vi "save_file.vi"(4 "offset":dbl, 5 "write OME header? (T)":bool=TRUE, 6 "multiplication factor":dbl=1.0, 7 "path":path, 8 "error in (no error)":errorcluster, 10 "ImageCollection in":refnum<class "ImageCollection.lvclass">, 11 "DataCollectionDL090215 in":refnum<class "DataCollectionMG091001IntrinsicImaging.lvclass">) -> (0 "error out":errorcluster, 3 "DataCollectionDL090215 out":refnum<class "DataCollectionMG091001IntrinsicImaging.lvclass">)   [LabVIEW 2010, in "DataCollectionMG091001IntrinsicImaging.lvclass"]
uses:
  DataCollectionMG091001IntrinsicImaging.lvclass
  common/classes/ImageCollection/ImageCollection/ImageCollection.lvclass
  common/classes/Image/Image/target_format_enum.ctl
  common/classes/ImageCollection/ImageCollection/saving_parameters_cluster.ctl
  common/classes/XMLElement/XMLElement/XMLElement.lvclass
  common/classes/ImageCollection/ImageCollection/OME_parameters_cluster.ctl
  common/classes/ImageCollection/ImageCollection/dimension_order_enum.ctl
  common/classes/GenericComponent/GenericComponent/GenericComponent.lvclass
  common/classes/ErrorController/ErrorController/class_data.vi
  common/classes/ErrorController/ErrorController/ErrorController.lvclass
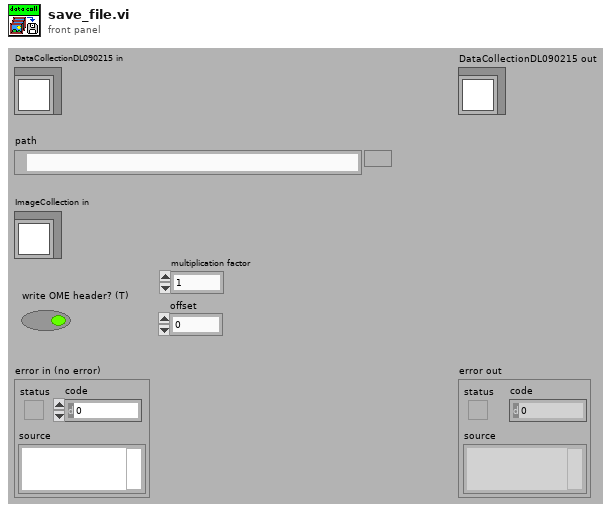
[diagram p1: front panel]
types:
  T1 = typedef "target_format_enum.ctl" = enum16{"don't force", "uint8", "uint16", "int16", "uint32", "int32", "single float"}
  T2 = typedef "ImageCollection.lvclass/saving_parameters_cluster.ctl" = cluster{"write OME header?":bool, "save as list file?":bool, "force format?":T1, "multiplication factor":dbl, "offset":dbl}
  T3 = typedef "dimension_order_enum.ctl" = enum16{"XYZCT", "XYZTC", "XYCTZ", "XYCZT", "XYTCZ", "XYTZC"}
  T4 = typedef "OME_parameters_cluster.ctl" = cluster{"image ID":string, "pixels ID":string, "dimension order":T3, "number of channels":i32}
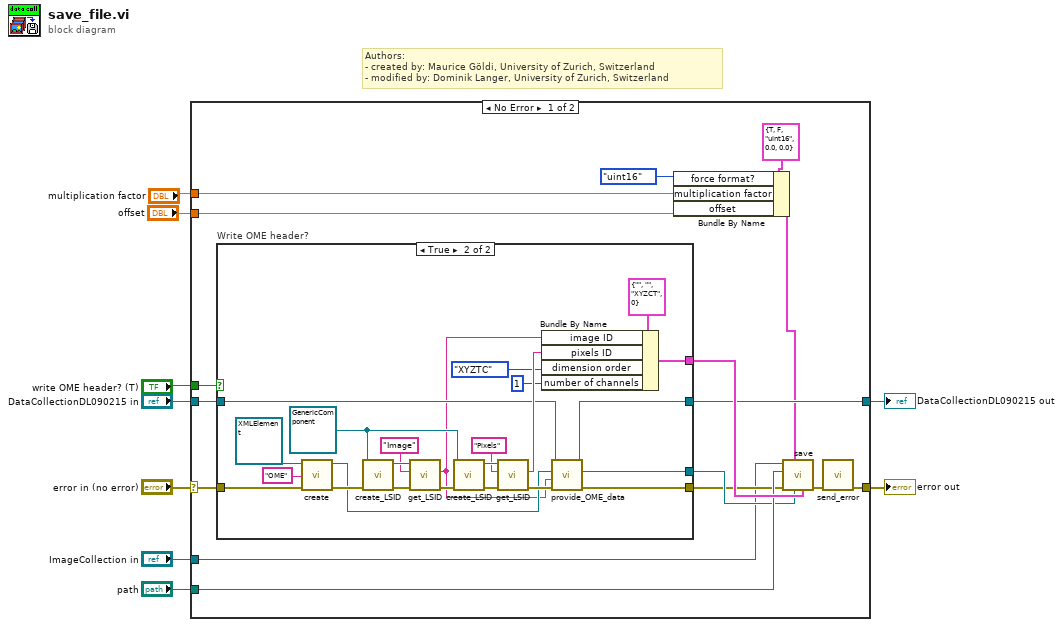
[diagram p0: block diagram]
diagram:
  # "Authors: \n- created by: Maurice Göldi, University of Zurich, Switzerland\n- modified by: Dominik Langer, University of Zurich, Switzerland"
  n1 = case shown="No Error" "error in (no error)" {
    selector: "error in (no error)" -> [w18 w53]
    tunnel: [w17 w53] -> w8
    tunnel: [w22 w52] -> w7
    tunnel: "DataCollectionDL090215 in" -> [w23 w52]
    tunnel: "ImageCollection in" -> [w15 _]
    tunnel: "path" -> [w24 _]
    tunnel: "write OME header? (T)" -> [w19 _]
    tunnel: "multiplication factor" -> [w11 _]
    tunnel: "offset" -> [w10 _]
    frame No Error {
      n2 = case "Write OME header?" shown="True" w19 {
        tunnel: w18 -> [w26 w50]
        tunnel: [_ w38] -> w25
        tunnel: w23 -> [w27 w33]
        tunnel: [w27 w32] -> w22
        tunnel: [_ w29] -> w21
        tunnel: [w26 w28] -> w20
        frame False {
        }
        frame True {
          w44 = refnum<class "GenericComponent.lvclass"> refnum ("GenericComponent.lvclass")
          n3 = call "create.vi"("error in (no error)"=w50, "name"="OME", "XMLElement in"=refnum<class "XMLElement.lvclass"> refnum ("XMLElement.lvclass")) -> ("error out"=w45:errorcluster, "XMLElement out"=w31:refnum<class "XMLElement.lvclass">)  [unwired: 7 in]
          n4 = call-dynamic "create_LSID.vi"("error in (no error)"=w45, "GenericPlugin in"=w44) -> ("error out"=w48:errorcluster, "GenericPlugin out"=w43:refnum<class "GenericComponent.lvclass">)  [unwired: 7 in, 1 out]
          n5 = call-dynamic "get_LSID.vi"("error in (no error)"=w48, "namespace"="Image", "GenericPlugin in"=w43) -> ("error out"=w47:errorcluster, "LSID (string)"=w30:string)  [unwired: 5 in, 2 out]
          n6 = call-dynamic "create_LSID.vi"("error in (no error)"=w47, "GenericPlugin in"=w44) -> ("error out"=w46:errorcluster, "GenericPlugin out"=w42:refnum<class "GenericComponent.lvclass">)  [unwired: 7 in, 1 out]
          n7 = call-dynamic "get_LSID.vi"("error in (no error)"=w46, "namespace"="Pixels", "GenericPlugin in"=w42) -> ("error out"=w34:errorcluster, "LSID (string)"=w37:string)  [unwired: 5 in, 2 out]
          n8 = Bundle By Name(cluster=T4 {"image ID"="", "pixels ID"="", "dimension order"=enum."XYZCT", "number of channels"=0} ("OME parameters"), "image ID"=w30, "pixels ID"=w37, "dimension order"=dimension_order_enum."XYZTC", "number of channels"=1) -> (w38:T4)
          n9 = call-dynamic "provide_OME_data.vi"("error in (no error)"=w34, "image ID"=w30, "OME element in"=w31, "DataCollectionDL091104Scaffold in"=w33) -> ("error out"=w28:errorcluster, "OME element out"=w29:refnum<class "XMLElement.lvclass">, "DataCollectionDL091104Scaffold out"=w32:refnum<class "DataCollectionMG091001IntrinsicImaging.lvclass">)  [unwired: 5 in]
        }
      }
      n10 = Bundle By Name(cluster=T2 {"write OME header?"=TRUE, "save as list file?"=FALSE, "force format?"=enum."uint16", "multiplication factor"=0.0, "offset"=0.0} ("saving parameters"), "force format?"=target_format_enum."uint16", "multiplication factor"=w11, "offset"=w10) -> (w13:T2)
      n11 = call "save.vi"("OME parameters"=w25, "OME XMLElement"=w21, "saving parameters"=w13, "error in (no error)"=w20, "path"=w24, "ImageCollection in"=w15) -> ("error out"=w16:errorcluster)  [unwired: 4 in, 1 out]
      n12 = call "send_error.vi"("error in (no error)"=w16) -> ("error out"=w17:errorcluster)  [unwired: 10 in]
    }
    frame Error {
    }
  }
  "error out" <- w8
  "DataCollectionDL090215 out" <- w7
